vi "ShiftArrElStringGen.vi"(8 "ErrorIn(No Error)":errorcluster caption="entrée d'erreur (pas d'erreur)", 9 "Index":i32, 10 "Dir(DownFalse)":bool, 11 "Array In":string[](array[string])) -> (0 "sortie d'erreur":errorcluster, 2 "NewIndex":i32, 3 "Array Out":string[](array[string]))   [LabVIEW 2019]
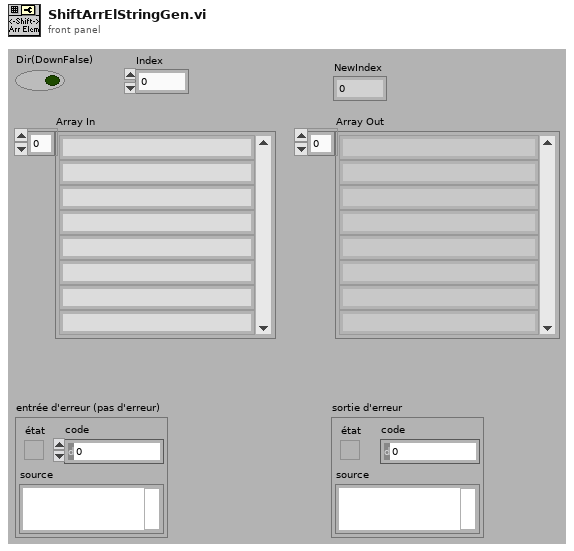
[diagram p1: front panel]
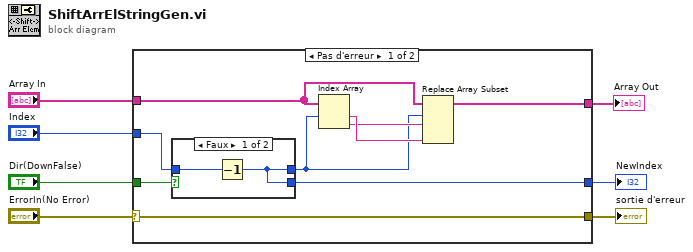
[diagram p0: block diagram]
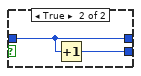
[diagram p2: hidden frame]
diagram:
  n1 = case shown="Pas d'erreur" "ErrorIn(No Error)" {
    selector: "ErrorIn(No Error)" -> [w16 w23]
    tunnel: [w16 w23] -> w6
    tunnel: "Array In" -> [w12 w22]
    tunnel: [w13 w22] -> w4
    tunnel: "Dir(DownFalse)" -> [w15 _]
    tunnel: "Index" -> [w14 w21]
    tunnel: [w8 w21] -> w1
    frame No Error {
      n2 = case shown="Faux" w15 {
        tunnel: w14 -> [w18 w20]
        tunnel: [w17 w20] -> w9
        tunnel: [w17 w19] -> w8
        frame False {
          n3 = Decrement(x=w18) -> (x-1=w17:i32)
        }
        frame True {
          n4 = Increment(x=w20) -> (x+1=w19:i32)
        }
      }
      n5 = Index Array(array=w12, index #1=w9) -> (element #1=w11:string, element #2=w10:string)  [unwired: 1 in]
      n6 = Replace Array Subset(array=w12, new element #1=w10, index #1=w9, new element #2=w11) -> (w13:string[])  [unwired: 1 in]
    }
    frame Error {
    }
  }
  "sortie d'erreur" <- w6
  "Array Out" <- w4
  "NewIndex" <- w1
